vi "xeva-setTemperature.vi"(3 "error in (no error)":errorcluster, 4 "xeva-temperature":dbl, 5 "xeva-camref":T1) -> (0 "error out":errorcluster, 1 "xeva-temperatureSP-ok":bool)   [LabVIEW 2015]
uses:
  <vilib>/Xenics Infrared Solutions/Xeneth LabVIEW API/VIs/Controls/Camara.ctl
  <vilib>/Xenics Infrared Solutions/Xeneth LabVIEW API/VIs/Property/XC Set Property Value L.vi
  <vilib>/Xenics Infrared Solutions/Xeneth LabVIEW API/Xeneth.lvlib
panel:
  out "error status":bool[](array[boolean])
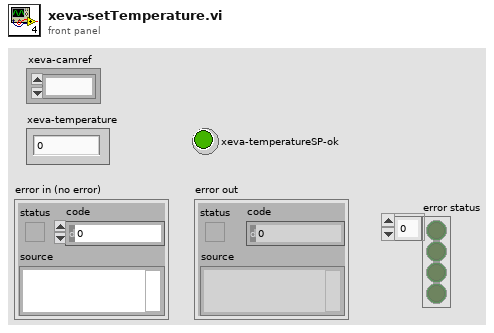
[diagram p1: front panel]
types:
  T1 = typedef "Xeneth.lvlib/Camara.ctl" = refnum<k1>
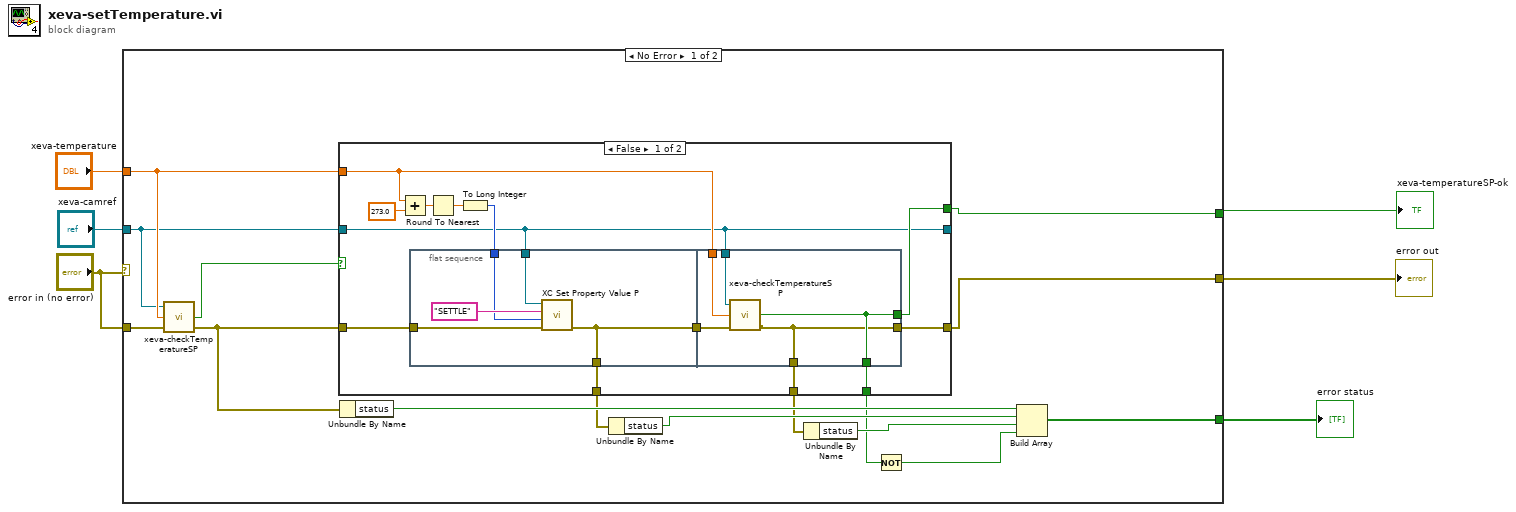
[diagram p0: block diagram]
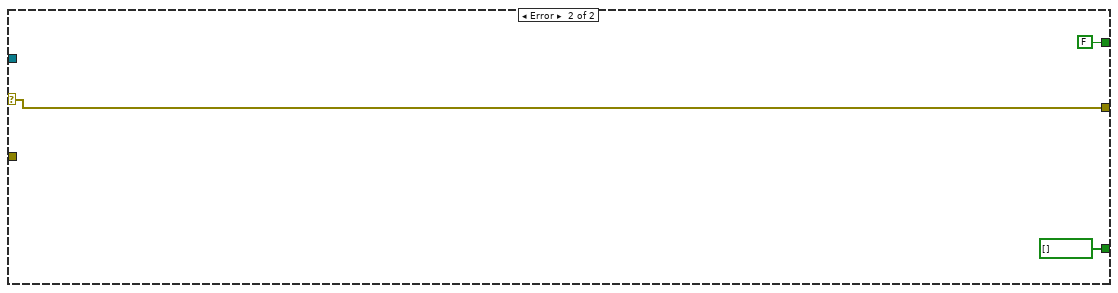
[diagram p3: hidden frame]
diagram:
  n1 = case shown="No Error" "error in (no error)" {
    selector: "error in (no error)" -> [_ w50]
    tunnel: "xeva-camref" -> [w7 _]
    tunnel: [w21 FALSE ("xeneth-temperatureSP-ok")] -> w5
    tunnel: "error in (no error)" -> [w20 _]
    tunnel: "xeva-temperature" -> [w19 _]
    tunnel: [w17 w50] -> w3
    tunnel: [w8 bool[] []] -> w1
    frame No Error {
      n2 = call "xeva-checkTemperatureSP.vi"("error in (no error)"=w20, "xeva-temperature"=w19, "xeva-camref"=w7) -> ("error out"=w16:errorcluster, "xeva-temperatureSP-ok"=w18:bool)  [unwired: 1 in]
      n3 = case shown="False" w18 {
        selector: w18 -> [_ w45]
        tunnel: [w27 w46] -> w17
        tunnel: w16 -> [w23 w46]
        tunnel: w7 -> [w28 w47]
        tunnel: w19 -> [w29 _]
        tunnel: [w30 w45] -> w21
        tunnel: [w28 w47] -> _
        tunnel: [w26 w45] -> w9
        tunnel: [w25 w46] -> w13
        tunnel: [w24 w46] -> w12
        frame False {
          n4 = Add(x=w29, y=273.0 ("x")) -> (x+y=w34:dbl)
          n5 = flat-sequence {
            tunnel: w32 -> [w38]
            tunnel: w28 -> [w37]
            tunnel: [w35] -> w25
            tunnel: w23 -> [w36]
            tunnel: [w35] -> w22
            tunnel: [w42] -> w30
            tunnel: w29 -> [w44]
            tunnel: w28 -> [w43]
            tunnel: [w41] -> w27
            tunnel: [w42] -> w26
            tunnel: [w41] -> w24
            tunnel: w22 -> [w40]
            frame #0 {
              n6 = call-poly <vilib>:"XC Set Property Value P.vi"("error in (no error)"=w36, "lValue"=w38, "pPrp"="SETTLE", "Cam Ref"=w37) -> ("error out"=w35:errorcluster)  [unwired: 6 in, 1 out]
            }
            frame #1 {
              n7 = call "xeva-checkTemperatureSP.vi"("error in (no error)"=w40, "xeva-temperature"=w44, "xeva-camref"=w43) -> ("error out"=w41:errorcluster, "xeva-temperatureSP-ok"=w42:bool)  [unwired: 1 in]
            }
          }
          n8 = Round To Nearest(number=w34) -> (nearest integer value=w33:dbl)
          n9 = To Long Integer(number=w33) -> (32bit integer=w32:i32)
        }
        frame True {
        }
      }
      n10 = Unbundle By Name(w16) -> ("status"=w14:bool)
      n11 = Unbundle By Name(w13) -> ("status"=w15:bool)
      n12 = Unbundle By Name(w12) -> ("status"=w11:bool)
      n13 = Not(x=w9) -> (.not. x?=w10:bool)
      n14 = Build Array(w14, w15, w11, w10) -> (w8:bool[])
    }
    frame Error {
    }
  }
  "error out" <- w3
  "xeva-temperatureSP-ok" <- w5
  "error status" <- w1
